vi "TCP communication_target.vi"(7 "TCP command":T1(ring), 8 "error in":errorcluster, 10 "timeout ms":i32=25000, 11 "Data in":string[](array[string])) -> (0 "error out":errorcluster, 2 "data out":string)   [LabVIEW 2011]
panel:
  in  "remote port":u16=6340
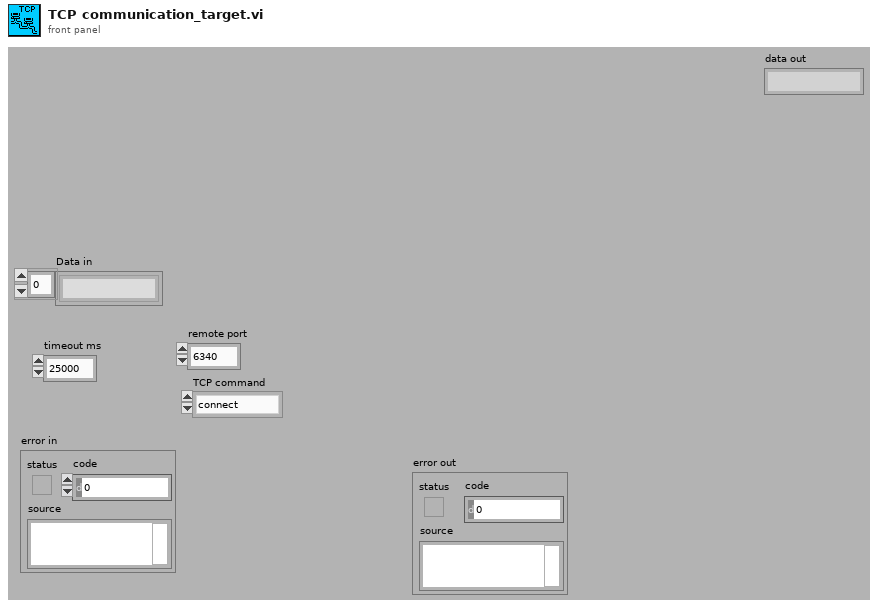
[diagram p1: front panel]
types:
  T1 = enum16{"connect", "receive data", "send data", "data transfer", "close"}
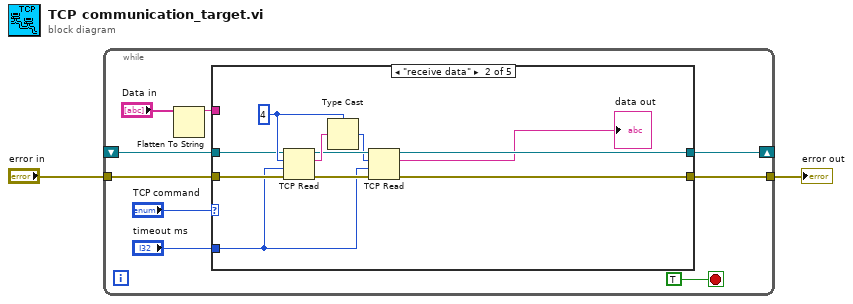
[diagram p0: block diagram]
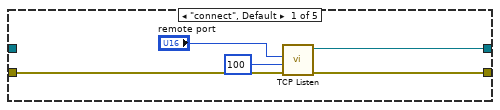
[diagram p2: hidden frame]
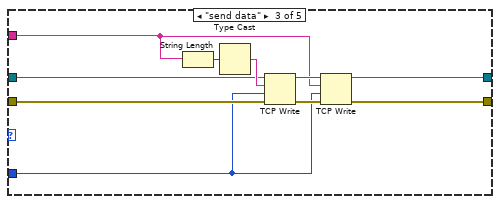
[diagram p3: hidden frame]
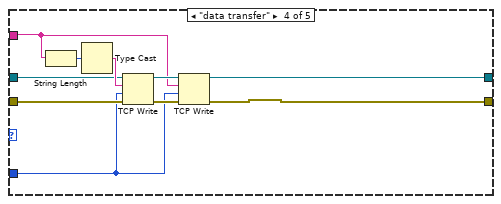
[diagram p4: hidden frame]
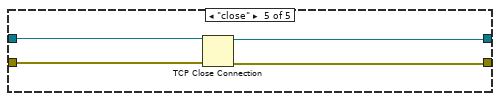
[diagram p5: hidden frame]
diagram:
  n1 = while {
    shift-right: [w11] -> _
    shift-left: _ -> [w9]
    tunnel: "error in" -> [w8]
    tunnel: [w7] -> w1
    stop <- TRUE stop-if-true
    n2 = Flatten To String(anything="Data in") -> (data string=w4:string)  [unwired: 3 in, 2 out]
    n3 = case shown="\"receive data\"" "TCP command" {
      tunnel: [w14 w21 w31 w39 w48] -> w11
      tunnel: w9 -> [_ w22 w32 w43 w49]
      tunnel: w8 -> [w12 w20 w29 w42 w51]
      tunnel: [w13 w18 w30 w38 w50] -> w7
      tunnel: w4 -> [_ _ w33 w41 _]
      tunnel: "timeout ms" -> [_ w19 w28 w40 _]
      frame "connect", Default {
        n4 = call <vilib>:"TCP Listen.vi"("error in (no error)"=w12, "timeout ms (wait forever: -1)"=100 ("timeout ms (60000)"), "port"="remote port") -> ("error out"=w13:errorcluster, "connection ID"=w14:refnum<k5>)  [unwired: 4 in, 3 out]
      }
      frame "receive data" {
        w23 = 4
        n5 = TCP Read(connection ID=w22, bytes to read=w23, error in (no error)=w20, 9:w19) -> (connection ID out=w26:refnum<k5>, data out=w27:string, error out=w25:errorcluster)  [unwired: 1 in]
        n6 = Type Cast(type=w23, x=w27) -> (*(type *) &x=w24:i32)
        n7 = TCP Read(connection ID=w26, bytes to read=w24, error in (no error)=w25, 9:w19) -> (connection ID out=w21:refnum<k5>, data out=→"data out":string, error out=w18:errorcluster)  [unwired: 1 in]
      }
      frame "send data" {
        n8 = String Length(string=w33) -> (length=w35:i32)
        n9 = Type Cast(x=w35) -> (*(type *) &x=w34:string)  [unwired: 1 in]
        n10 = TCP Write(connection ID=w32, data in=w34, error in (no error)=w29, 9:w28) -> (connection ID out=w37:refnum<k5>, error out=w36:errorcluster)  [unwired: 1 out]
        n11 = TCP Write(connection ID=w37, data in=w33, error in (no error)=w36, 9:w28) -> (connection ID out=w31:refnum<k5>, error out=w30:errorcluster)  [unwired: 1 out]
      }
      frame "data transfer" {
        n12 = String Length(string=w41) -> (length=w45:i32)
        n13 = Type Cast(x=w45) -> (*(type *) &x=w44:string)  [unwired: 1 in]
        n14 = TCP Write(connection ID=w43, data in=w44, error in (no error)=w42, 9:w40) -> (connection ID out=w47:refnum<k5>, error out=w46:errorcluster)  [unwired: 1 out]
        n15 = TCP Write(connection ID=w47, data in=w41, error in (no error)=w46, 9:w40) -> (connection ID out=w39:refnum<k5>, error out=w38:errorcluster)  [unwired: 1 out]
      }
      frame "close" {
        n16 = TCP Close Connection(connection ID=w49, error in (no error)=w51) -> (connection ID out=w48:refnum<k5>, error out=w50:errorcluster)  [unwired: 1 in]
      }
    }
  }
  "error out" <- w1
